vi "Variant Metadata.vi"(8 "error in (no error)":errorcluster, 11 "Variant":variant) -> (0 "error out":errorcluster, 2 "Treat As Array":bool, 3 "Name":string)   [LabVIEW 2020, in "JKI JSON Serialization.lvlib" / "JSON Serializer.lvclass"]
uses:
  JSON Serializer.lvclass
  JSON Serializer.lvclass/JSON Serializer.ctl
  <vilib>/Utility/Data Type/NI_Data Type.lvlib
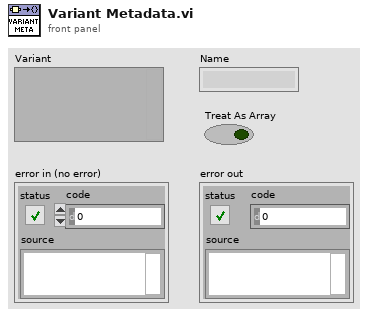
[diagram p1: front panel]
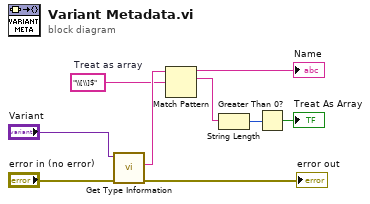
[diagram p0: block diagram]
diagram:
  w4 = "\\[\\]$"  # Treat as array
  n1 = call <vilib>:"Get Type Information.vi"("error in (no error)"="error in (no error)", "variant"="Variant") -> ("error out"=→"error out":errorcluster, "name"=w5:string)  [unwired: 5 in, 3 out]
  n2 = Match Pattern(string=w5, regular expression=w4) -> (before substring=→"Name":string, match substring=w6:string)  [unwired: 1 in, 2 out]
  n3 = String Length(string=w6) -> (length=w7:i32)
  n4 = Greater Than 0?(x=w7) -> (x > 0?=→"Treat As Array":bool)
